vi "get vi description.vi"(8 "error in (no error)":errorcluster, 11 "Description":string) -> (0 "error out":errorcluster, 3 "String":string)   [LabVIEW 2025, in "Scripting Server.lvlib" / "Tools.lvlib"]
uses:
  Tools.lvlib
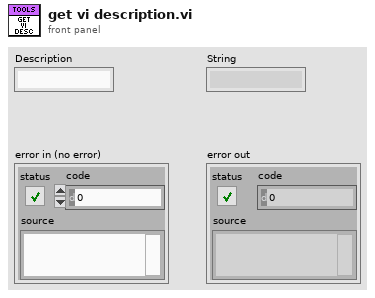
[diagram p1: front panel]
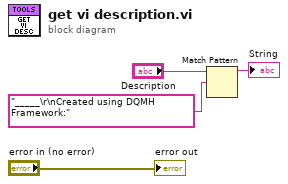
[diagram p0: block diagram]
diagram:
  n1 = Match Pattern(string="Description", regular expression="_____\r\nCreated using DQMH Framework:") -> (before substring=→"String":string)  [unwired: 1 in, 3 out]
  "error out" <- "error in (no error)"
